vi "Get LeafNodes.vi"(8 "error in (no error)":errorcluster caption="错误输入（无错误）", 11 "PanelLinkNode 输入":refnum<class "PanelLinkNode.lvclass"> caption="DNL_LabVIEW Object in") -> (0 "error out":errorcluster caption="错误输出", 2 "DataNode[]":refnum<data-value>[](array[refnum]), 3 "PanelLinkNode 输出":refnum<class "PanelLinkNode.lvclass"> caption="DNL_LabVIEW Object out")   [LabVIEW 2013, in "PanelLinkNode.lvclass"]
uses:
  PanelLinkNode.lvclass
  PanelObject/PanelObject.lvclass
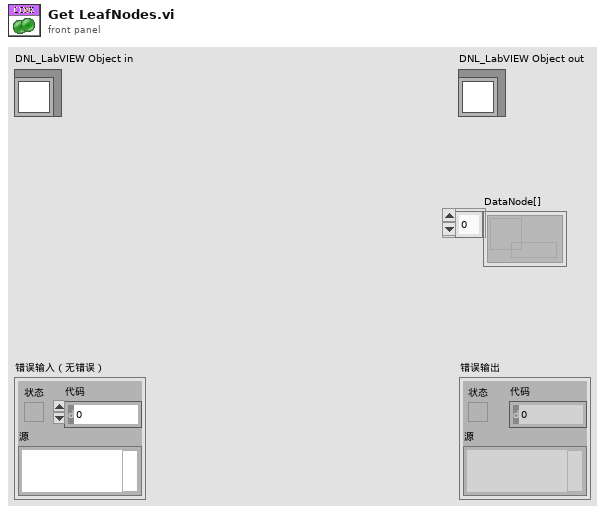
[diagram p1: front panel]
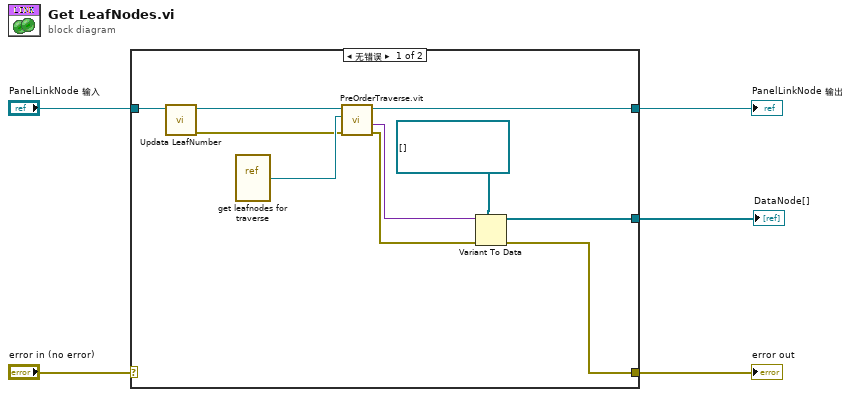
[diagram p0: block diagram]
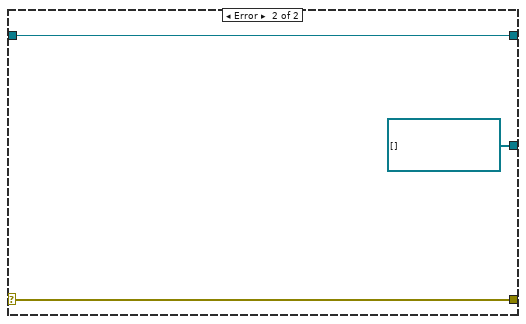
[diagram p2: hidden frame]
diagram:
  n1 = case shown="无错误" "error in (no error)" {
    selector: "error in (no error)" -> [_ w18]
    tunnel: [w6 w18] -> w4
    tunnel: [w13 w17] -> w2
    tunnel: "PanelLinkNode 输入" -> [w11 w17]
    tunnel: [w7 refnum<data-value>[] [] ("Data out")] -> w1
    frame No Error {
      n2 = call-dynamic "Updata LeafNumber.vi"("PanelLinkNode 输入"=w11) -> ("error out"=w9:errorcluster, "PanelLinkNode 输出"=w10:refnum<class "PanelLinkNode.lvclass">)  [unwired: 8 in, 1 out]
      n3 = vi-ref "get leafnodes for traverse.vi"() -> (w12:refnum<vi>)
      n4 = call-dynamic "PreOrderTraverse.vit"("error in"=w9, "vi reference"=w12, "PanelLinkNode 输入"=w10) -> ("error out"=w8:errorcluster, "Data out"=w15:variant, "PanelLinkNode 输出"=w13:refnum<class "PanelLinkNode.lvclass">)  [unwired: 5 in, 1 out]
      n5 = Variant To Data(error in=w8, type=refnum<data-value>[] [] ("Data out"), Variant=w15) -> (data=w7:refnum<data-value>[], error out=w6:errorcluster)
    }
    frame Error {
    }
  }
  "error out" <- w4
  "PanelLinkNode 输出" <- w2
  "DataNode[]" <- w1
